vi "FindLatestFile.vi"(7 "Check Type":T1, 9 "Contents":T3[](array[typedef])) -> (2 "Found":bool, 4 "Latest runtime":T3, 5 "Version":T2)   [LabVIEW 2014, in "GitHub API.lvlib"]
uses:
  GitHub API.lvlib
  TypeDefs/GitHubContents_TD.ctl
  RasPi_Services/Download/RuntimeVersion.ctl
  TypeDefs/GitHubCheckTypeTD.ctl
  RasPi_Services/Download/RasPiDownloader.lvlib
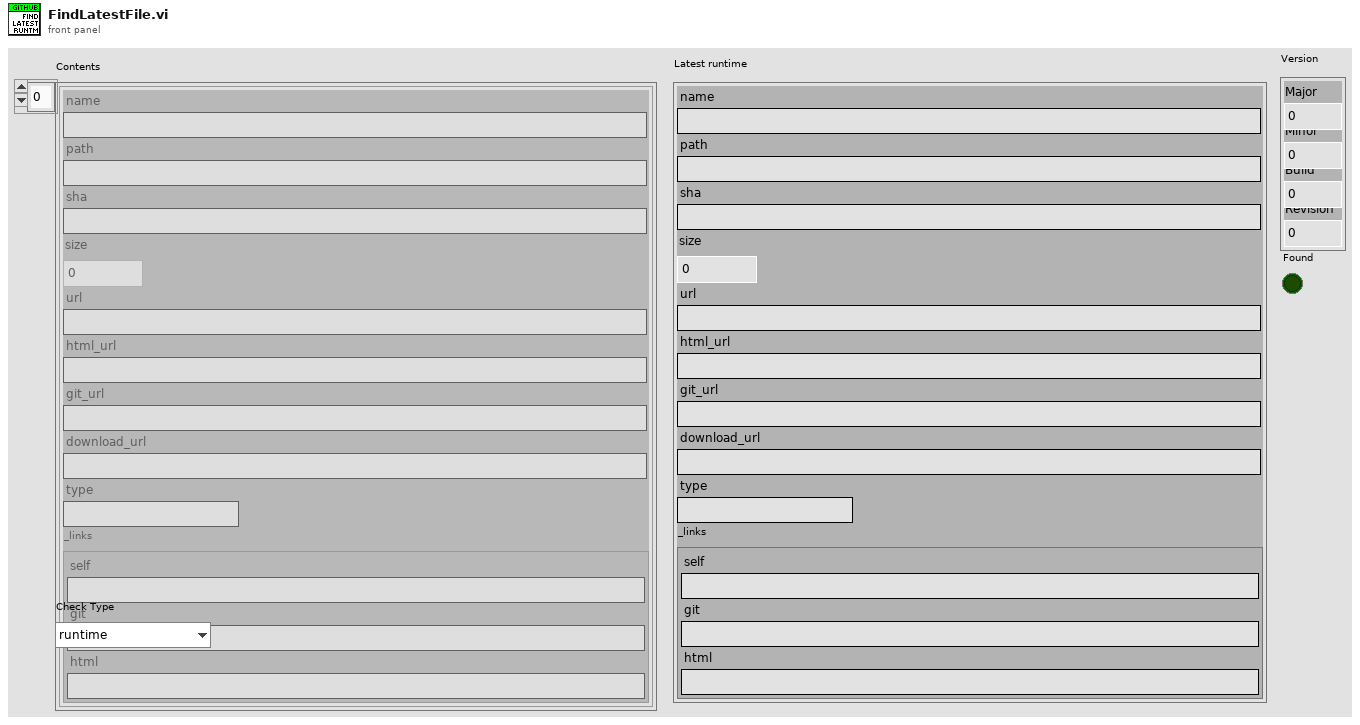
[diagram p1: front panel]
types:
  T1 = typedef "GitHub API.lvlib/GitHubCheckTypeTD.ctl" = enum16{"runtime", "VIPM Home Version", "VIPM Standard Version"}
  T2 = typedef "RasPiDownloader.lvlib/RuntimeVersion.ctl" = cluster{"Major":i32, "Minor":i32, "Build":i32, "Revision":i32}
  T3 = typedef "GitHub API.lvlib/GitHubContents_TD.ctl" = cluster{"name":string, "path":string, "sha":string, "size":dbl, "url":string, "html_url":string, "git_url":string, "download_url":string, "type":string, "_links":cluster{"self":string, "git":string, "html":string}}
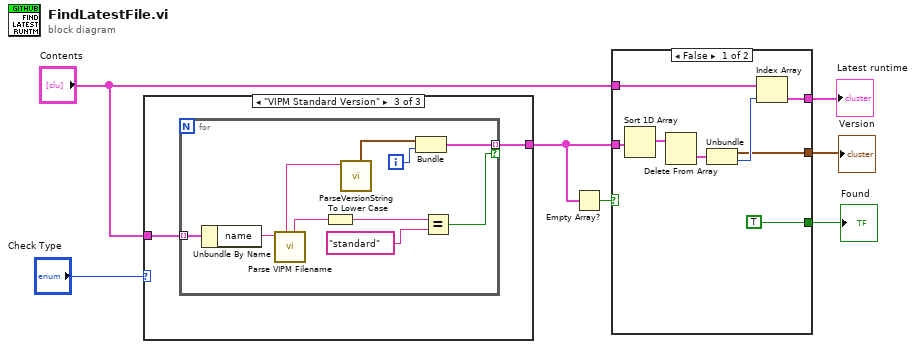
[diagram p0: block diagram]
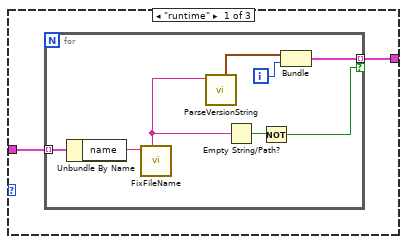
[diagram p2: hidden frame]
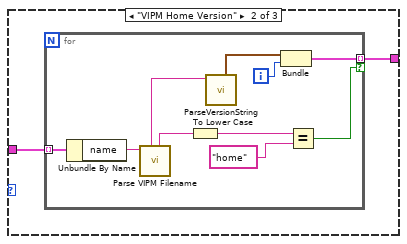
[diagram p3: hidden frame]
diagram:
  n1 = case shown="\"VIPM Standard Version\"" "Check Type" {
    tunnel: [w9 w19 w31] -> w7
    tunnel: "Contents" -> [w8 w18 w30]
    frame "runtime" {
      n2 = for {
        tunnel: w8 -> [w17] mode=indexing
        tunnel: [w14] -> w9 mode=indexing if=w12
        i -> [w10]
        n3 = Unbundle By Name(w17) -> ("name"=w16:string)
        n4 = call "FixFileName.vi"("Filename"=w16) -> ("version"=w15:string)  [unwired: 7 in, 1 out]
        n5 = call "ParseVersionString.vi"("version string"=w15) -> ("Version"=w11:T2)  [unwired: 7 in, 1 out]
        n6 = Empty String/Path?(string/path=w15) -> (empty?=w13:bool)
        n7 = Not(x=w13) -> (.not. x?=w12:bool)
        n8 = Bundle("Version"=w11, w10) -> (w14:cluster{"Version":T2, i32})  [unwired: 1 in]
      }
    }
    frame "VIPM Home Version" {
      n9 = for {
        tunnel: w18 -> [w29] mode=indexing
        tunnel: [w28] -> w19 mode=indexing if=w21
        i -> [w26]
        n10 = Unbundle By Name(w29) -> ("name"=w25:string)
        n11 = call "Parse VIPM Filename.vi"("Filename"=w25) -> ("edition"=w23:string, "version"=w24:string)  [unwired: 7 in]
        n12 = To Lower Case(string=w23) -> (all lower case string=w22:string)
        n13 = call "ParseVersionString.vi"("version string"=w24) -> ("Version"=w27:T2)  [unwired: 7 in, 1 out]
        n14 = Bundle("Version"=w27, w26) -> (w28:cluster{"Version":T2, i32})  [unwired: 1 in]
        n15 = Equal?(x=w22, y="home") -> (x = y?=w21:bool)
      }
    }
    frame "VIPM Standard Version" {
      n16 = for {
        tunnel: w30 -> [w41] mode=indexing
        tunnel: [w40] -> w31 mode=indexing if=w33
        i -> [w38]
        n17 = Unbundle By Name(w41) -> ("name"=w37:string)
        n18 = call "Parse VIPM Filename.vi"("Filename"=w37) -> ("edition"=w35:string, "version"=w36:string)  [unwired: 7 in]
        n19 = To Lower Case(string=w35) -> (all lower case string=w34:string)
        n20 = call "ParseVersionString.vi"("version string"=w36) -> ("Version"=w39:T2)  [unwired: 7 in, 1 out]
        n21 = Bundle("Version"=w39, w38) -> (w40:cluster{"Version":T2, i32})  [unwired: 1 in]
        n22 = Equal?(x=w34, y="standard") -> (x = y?=w33:bool)
      }
    }
  }
  n23 = Empty Array?(array=w7) -> (empty?=w6:bool)
  n24 = case shown="False" w6 {
    tunnel: w7 -> [w49 _]
    tunnel: "Contents" -> [w46 _]
    tunnel: [w45 _] -> w4
    tunnel: [TRUE _] -> w3
    tunnel: [w42 _] -> w2
    frame False {
      n25 = Sort 1D Array(array=w49) -> (sorted array=w48:cluster{"Version":T2, i32}[])
      n26 = Delete From Array(array=w48) -> (deleted portion=w47:cluster{"Version":T2, i32})  [unwired: 2 in, 1 out]
      n27 = Unbundle(w47) -> ("Version"=w42:T2, w44:i32)
      n28 = Index Array(array=w46, index=w44) -> (element=w45:T3)
    }
    frame True {
    }
  }
  "Latest runtime" <- w4
  "Found" <- w3
  "Version" <- w2
